vi "S2C_Shared_Proc_ShowProcess.vi"(8 "Error In":errorcluster, 11 "ProcessName":string) -> (0 "Error Out":errorcluster)   [LabVIEW 2015]
doc: "Displays the Fornax communication process VI."
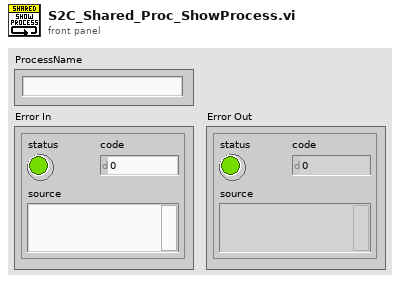
[diagram p1: front panel]
types:
  T1 = enum32{"Invalid", "Standard", "Closed", "Hidden", "Minimized", "Maximized"}
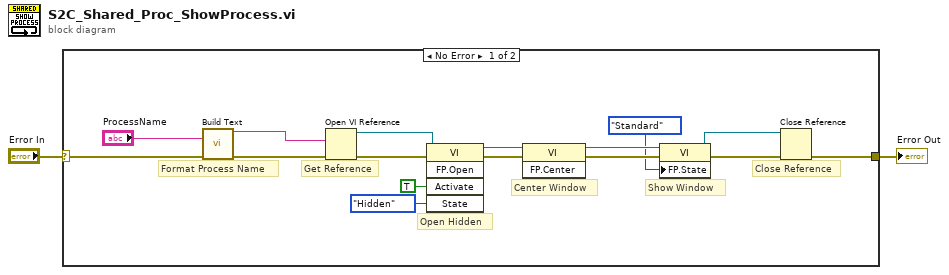
[diagram p0: block diagram]
diagram:
  n1 = case shown="No Error" "Error In" {
    selector: "Error In" -> [w6 w19]
    tunnel: [w18 w19] -> w1
    frame No Error {
      # "Format Process Name"
      # "Close Reference"
      # "Show Window"
      # "Center Window"
      # "Open Hidden"
      # "Get Reference"
      n2 = call "Build Text"("Driver"="ProcessName", "error in (no error)"=w6) -> ("Result"=w4:string, "error out"=w5:errorcluster)  [unwired: 12 in]
      n3 = Open VI Reference(vi path=w4, error in (no error)=w5) -> (vi reference=w14:refnum<vi>, error out=w15:errorcluster)  [unwired: 4 in]
      n4 = invoke class="VI" method="FP.Open"(reference=w14, error in=w15, "Activate"=TRUE ("Activate?"), "State"=T1."Hidden") -> (reference out=w12:refnum<vi>, error out=w13:errorcluster)  [unwired: 1 in, 3 out]
      n5 = invoke class="VI" method="FP.Center"(reference=w12, error in=w13) -> (reference out=w10:refnum<vi>, error out=w11:errorcluster)  [unwired: 1 in, 1 out]
      n6 = property class="VI"(reference=w10, error in=w11, "FP.State"=T1."Standard" ("Front Panel Window:State")) -> (reference out=w7:refnum<vi>, error out=w9:errorcluster)
      n7 = Close Reference(reference=w7, error in (no error)=w9) -> (error out=w18:errorcluster)
    }
    frame Error {
    }
  }
  "Error Out" <- w1
